vi "DAQmx有限采样.vi"() -> ()   [LabVIEW 2010]
uses:
  <vilib>/DAQmx/read.llb/DAQmx Read.vi
  <vilib>/DAQmx/read.llb/DAQmx Read (Analog 1D DBL 1Chan NSamp).vi
  <vilib>/DAQmx/create/channels.llb/DAQmx Create Channel (AI-Voltage-Basic).vi
  <vilib>/DAQmx/configure/timing.llb/DAQmx Timing (Sample Clock).vi
  <vilib>/daqmx/miscellaneous.llb/DAQmx Fill In Error Info.vi
panel:
  out "data":dbl[](graph)
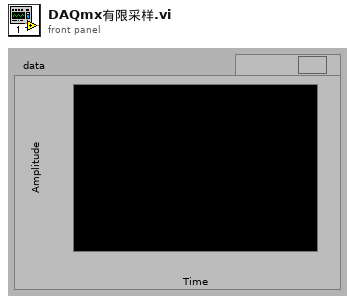
[diagram p1: front panel]
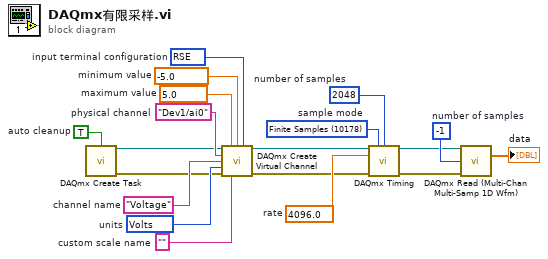
[diagram p0: block diagram]
diagram:
  w17 = 10178 items=["Finite Samples"=10178, "Continuous Samples"=10123]  # sample mode
  w16 = 2048  # number of samples
  w15 = 4096.0  # rate
  w14 = 10083 items=["default"=-1, "differential"=10106, "RSE"=10083, "NRSE"=10078]  # input terminal configuration
  w13 = 10348 items=["Volts"=10348, "From Custom Scale"=10065]  # units
  w12 = "Voltage"  # channel name
  w9 = ""  # custom scale name
  w8 = -5.0  # minimum value
  w7 = 5.0  # maximum value
  w6 = "Dev1/ai0"  # physical channel
  w5 = TRUE  # auto cleanup
  w18 = -1  # number of samples
  n1 = call <vilib>:"DAQmx Create Task.vi"("auto cleanup"=w5) -> ("task out"=w4:refnum<k21>, "error out"=w3:errorcluster)  [unwired: 13 in]
  n2 = call-poly <vilib>:"DAQmx Create Virtual Channel.vi"("task in"=w4, "maximum value"=w7, "minimum value"=w8, "input terminal configuration"=w14, "physical channels"=w6, "name to assign"=w12, "units"=w13, "error in"=w3, "custom scale name"=w9) -> ("task out"=w10:refnum<k21>, "error out"=w11:errorcluster)  [unwired: 5 in]
  n3 = call-poly <vilib>:"DAQmx Timing.vi"("task/channels in"=w10, "sample mode"=w17, "samples per channel"=w16, "rate"=w15, "error in"=w11) -> ("task out"=w2:refnum<k21>, "error out"=w1:errorcluster)  [unwired: 9 in]
  n4 = call-poly "DAQmx Read (Multi-Chan Multi-Samp 1D Wfm).vi"("task/channels in"=w2, "number of samples per channel"=w18, "error in"=w1) -> ("data"=→"data":dbl[])  [unwired: 10 in, 2 out]
